vi "PointToRoi.vi"(7 "Director":enum16{"Left", "Top", "Right", "Bottom"}(ring), 8 "error in (no error)":errorcluster, 9 "ROISize":cluster{"Width":dbl, "Height":dbl}, 10 "r":dbl, 11 "Point":T1 {"Y" format="%.2f"; "X" format="%.2f"}) -> (0 "error out":errorcluster, 3 "ROI Descriptor":T2 {"Contours"."Type" items=["No Selection", "Point", "Line", "Rectangle", "Oval", "Polygon", "Freehand Region", "Annulus", "Unused2", "Unused3", "Broken Line", "Freehand Line", "Rotated Rectangle"]})   [LabVIEW 2015]
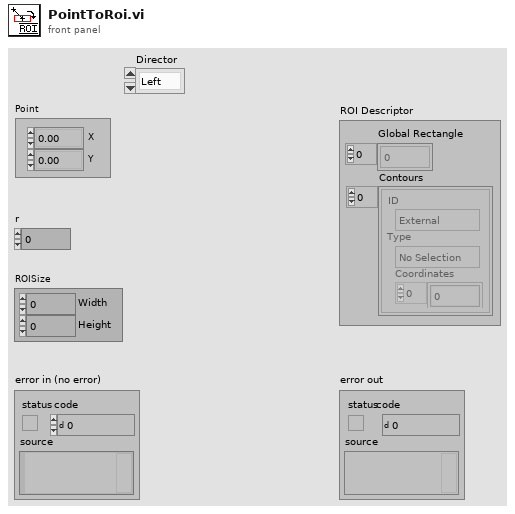
[diagram p1: front panel]
types:
  T1 = typedef "IMAQ Point" = cluster{"X":sgl, "Y":sgl}
  T2 = typedef "ROI Descriptor" = cluster{"Global Rectangle":i32[], "Contours":cluster{"ID":enum32{"External", "Internal"}, "Type":u32, "Coordinates":i32[]}[]}
  T3 = cluster{"ID":enum32{"External", "Internal"}, "Type":u32, i32[]}
  T4 = cluster{"ID":enum32{"External", "Internal"}, "Type":u32, i32[]}[]
  T5 = cluster{i32[], cluster{"ID":enum32{"External", "Internal"}, "Type":u32, i32[]}[]}
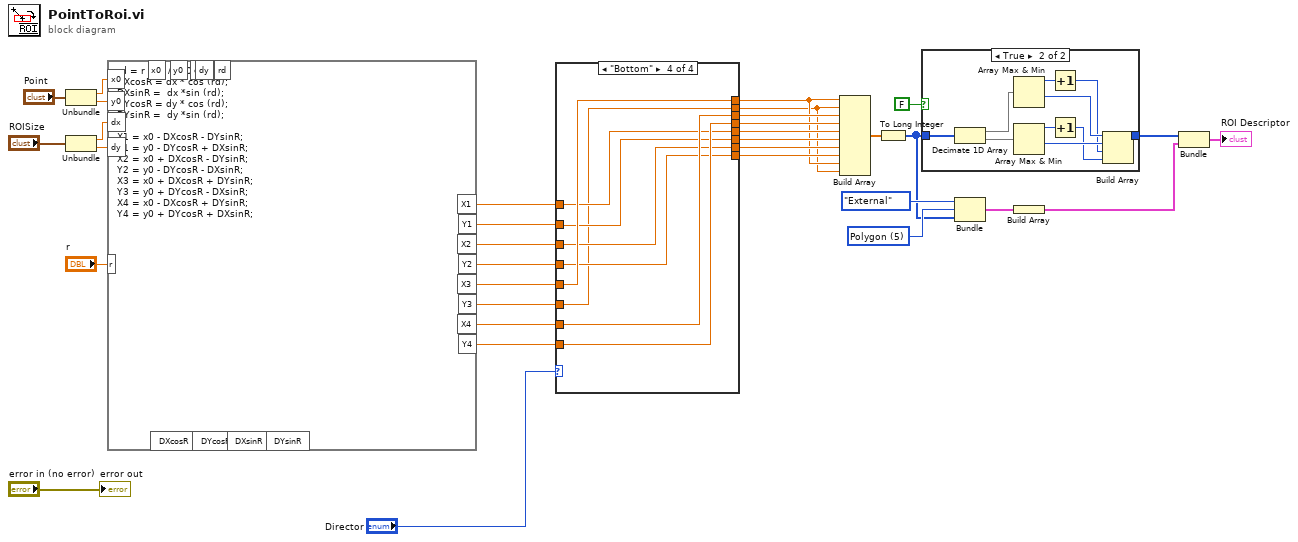
[diagram p0: block diagram]
diagram:
  w31 = u32 5 items=["No Selection", "Point", "Line", "Rectangle", "Oval", "Polygon", "Free", "Annulus", "Unused2", "Unused3", "Broken Line", "Free Hand Line", "Rotated Rectangle"] ("Type")
  n1 = Unbundle("Point") -> ("X"=w24:sgl, "Y"=w23:sgl)
  n2 = Unbundle("ROISize") -> ("Width"=w21:dbl, "Height"=w20:dbl)
  n3 = formula code="rd = r * pi / 180.0;\nDXcosR = dx * cos (rd);\nDXsinR =  dx *sin (rd);\nDYcosR = dy * cos (rd);\nDYsinR =  dy *sin (rd);\n\nX1 = x0 - DXcosR - DYsinR;\nY1 = y0 - DYcosR + DXsinR;\nX2 = x0 + DXcosR - DYsinR;\nY2 = y0 - DYcosR - DXsinR;\nX3 = x0 + DXcosR + DYsinR;\nY3 = y0 + DYcosR - DXsinR;\nX4 = x0 - DXcosR + DYsinR;\nY4 = y0 + DYcosR + DXsinR;"("r"="r", "x0"=w24, "y0"=w23, "dx"=w21, "dy"=w20) -> ("X1"=w17:dbl, "Y1"=w16:dbl, "X2"=w2:dbl, "Y2"=w15:dbl, "X3"=w14:dbl, "Y3"=w13:dbl, "X4"=w12:dbl, "Y4"=w11:dbl)  [unwired: 9 out]
  n4 = case shown="\"Bottom\"" "Director" {
    tunnel: w17 -> [w42 w50 w52 w63]
    tunnel: w16 -> [w41 w49 w51 w62]
    tunnel: w2 -> [w40 w48 w58 w61]
    tunnel: w15 -> [w39 w47 w57 w60]
    tunnel: w14 -> [w38 w46 w56 w66]
    tunnel: w13 -> [w37 w45 w55 w59]
    tunnel: w12 -> [w36 w44 w54 w65]
    tunnel: w11 -> [w35 w43 w53 w64]
    tunnel: [w36 w50 w58 w66] -> w4
    tunnel: [w35 w49 w57 w59] -> w3
    tunnel: [w42 w48 w56 w65] -> w10
    tunnel: [w41 w47 w55 w64] -> w9
    tunnel: [w40 w46 w54 w63] -> w8
    tunnel: [w39 w45 w53 w62] -> w7
    tunnel: [w38 w44 w52 w61] -> w6
    tunnel: [w37 w43 w51 w60] -> w5
    frame "Right", Default {
    }
    frame "Top" {
    }
    frame "Left" {
    }
    frame "Bottom" {
    }
  }
  n5 = Build Array(w4, w3, w10, w9, w8, w7, w6, w5, w4, w3) -> (w30:dbl[])
  n6 = To Long Integer(number=w30) -> (32bit integer=w29:i32[])
  n7 = case shown="True" FALSE {
    tunnel: w29 -> [w67 w73]
    tunnel: [w67 w72] -> w28
    frame False {
    }
    frame True {
      n8 = Decimate 1D Array(w73) -> (w70:i32[], w71:i32[])
      n9 = Array Max & Min(array=w70) -> (max value=w75:i32, min value=w77:i32)  [unwired: 2 out]
      n10 = Array Max & Min(array=w71) -> (max value=w74:i32, min value=w76:i32)  [unwired: 2 out]
      n11 = Increment(x=w75) -> (x+1=w69:i32)
      n12 = Increment(x=w74) -> (x+1=w68:i32)
      n13 = Build Array(w77, w76, w69, w68) -> (w72:i32[])
    }
  }
  n14 = Bundle("ID"=enum32{"External", "Internal"}."External", "Type"=w31, w29) -> (w33:T3)  [unwired: 1 out]
  n15 = Build Array(w33) -> (w34:T4)
  n16 = Bundle(w28, w34) -> (→"ROI Descriptor":T5)  [unwired: 1 out]
  "error out" <- "error in (no error)"
